vi "app_pktGen.vi"(11 "appended array":string[](array[string])) -> (3 "packets":string[](array[string]))   [LabVIEW 2014]
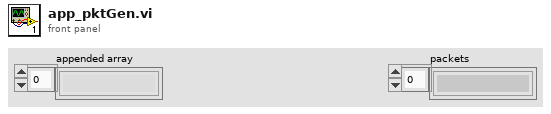
[diagram p1: front panel]
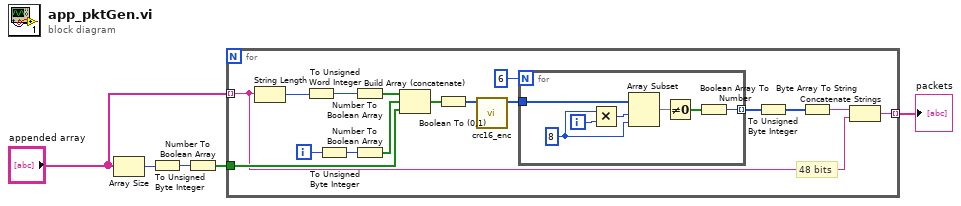
[diagram p0: block diagram]
diagram:
  n1 = Array Size(array="appended array") -> (size(s)=w4:i32)
  n2 = To Unsigned Byte Integer(number=w4) -> (unsigned 8bit integer=w3:u8)
  n3 = Number To Boolean Array(number=w3) -> (Boolean array=w2:bool[])
  n4 = for {
    tunnel: "appended array" -> [w7] mode=indexing
    tunnel: w2 -> [w15]
    tunnel: [w6] -> w1 mode=indexing
    i -> [w21]
    # "48 bits"
    n5 = String Length(string=w7) -> (length=w20:i32)
    n6 = To Unsigned Word Integer(number=w20) -> (unsigned 16bit integer=w19:u16)
    n7 = To Unsigned Byte Integer(number=w21) -> (unsigned 8bit integer=w18:u8)
    n8 = Number To Boolean Array(number=w19) -> (Boolean array=w17:bool[])
    n9 = Number To Boolean Array(number=w18) -> (Boolean array=w16:bool[])
    n10 = Build Array (concatenate)(w17, w16, w15) -> (w14:bool[])
    n11 = Boolean To (0,1)(Boolean=w14) -> (0, 1=w13:i16[])
    n12 = call "crc16_enc.vi"("bits"=w13) -> ("appended bits"=w12:i16[])  [unwired: 10 in]
    n13 = for {
      N: 6 -> [_]
      tunnel: w12 -> [w28]
      tunnel: [w22] -> w10 mode=indexing
      i -> [w27]
      w25 = 8 ("x")
      n14 = Multiply(x=w25, y=w27) -> (x*y=w26:i32)
      n15 = Array Subset(array=w28, index=w26, length=w25) -> (w24:i16[])
      n16 = Not Equal To 0?(x=w24) -> (x != 0?=w23:bool[])
      n17 = Boolean Array To Number(Boolean array=w23) -> (number=w22:u32)
    }
    n18 = To Unsigned Byte Integer(number=w10) -> (unsigned 8bit integer=w9:u8[])
    n19 = Byte Array To String(unsigned byte array=w9) -> (string=w8:string)
    n20 = Concatenate Strings(w8, w7) -> (w6:string)
  }
  "packets" <- w1
